vi "Read_func.vi"(8 "error in (no error)":errorcluster, 11 "Data Cluster in":T1) -> (0 "error out":errorcluster, 1 "bytes read":u32, 2 "read buffer":string, 3 "Data Cluster out":T1, 4 "Status":bool)   [LabVIEW 2017, in "FingerPrintMânager.lvlib"]
uses:
  Module Data--cluster.ctl
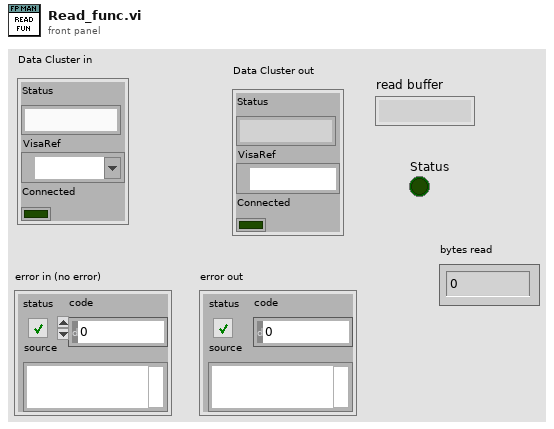
[diagram p1: front panel]
types:
  T1 = typedef "FingerPrintMânager.lvlib/Module Data--cluster.ctl" = cluster{"Status":string, "VisaRef":refnum<visa-resource-name>, "Connected":bool}
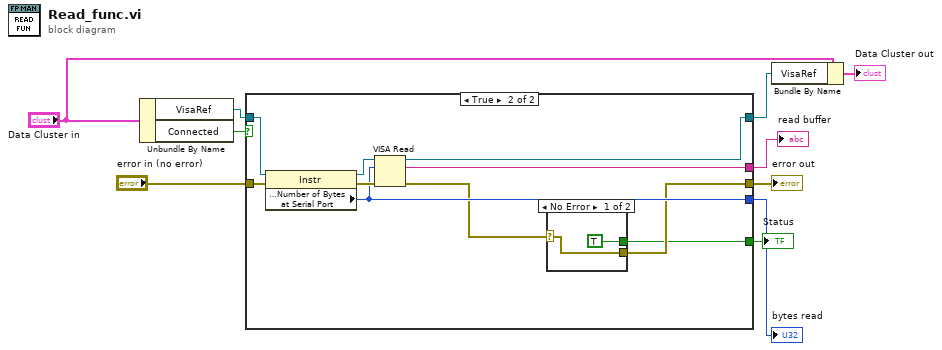
[diagram p0: block diagram]
diagram:
  n1 = Unbundle By Name("Data Cluster in") -> ("VisaRef"=w5:refnum<visa-resource-name>, "Connected"=w4:bool)
  n2 = case shown="True" w4 {
    tunnel: "error in (no error)" -> [w12 w17]
    tunnel: [w12 w14] -> w8
    tunnel: [w11 w18] -> w10
    tunnel: w5 -> [w11 w19]
    tunnel: [_ w20] -> w3
    tunnel: [_ w16] -> w2
    tunnel: [_ w13] -> w1
    frame False {
    }
    frame True {
      n3 = property class="Instr"(reference=w19, error in=w17) -> (reference out=w22:refnum<visa-resource-name>, error out=w21:errorcluster, "Serial Settings:Number of Bytes at Serial Port"=w20:u32)
      n4 = VISA Read(VISA resource name=w22, byte count=w20, error in (no error)=w21) -> (VISA resource name out=w18:refnum<visa-resource-name>, read buffer=w16:string, error out=w15:errorcluster)  [unwired: 1 out]
      n5 = case shown="No Error" w15 {
        selector: w15 -> [w24 w25]
        tunnel: [w24 w25] -> w14
        tunnel: [TRUE _] -> w13
        frame No Error {
        }
        frame Error {
        }
      }
    }
  }
  "error out" <- w8
  "bytes read" <- w3
  "read buffer" <- w2
  "Status" <- w1
  n6 = Bundle By Name(cluster="Data Cluster in", "VisaRef"=w10) -> (→"Data Cluster out":T1)
